vi "Create Upgrade Response.vi"(8 "error in (no error)":errorcluster, 10 "Sec-WebSocket-Key":string) -> (0 "error out":errorcluster, 2 "WebSocketUpgradeResponse":refnum<class "WebSocketUpgradeResponse.lvclass">)   [LabVIEW 2020, in "HTTP Server.lvlib" / "WebSocket Client.lvclass"]
uses:
  WebSocket Client.lvclass
  WebSocketUpgradeResponse/WebSocketUpgradeResponse.lvclass
  C:/dev/lv20CE/relink/lv-http-util/HTTP Utils/Response/Response.lvclass
  WebSocket Client.lvclass/WebSocket Client.ctl
  lv-http-util/HTTP Utils/Response/Response.lvclass
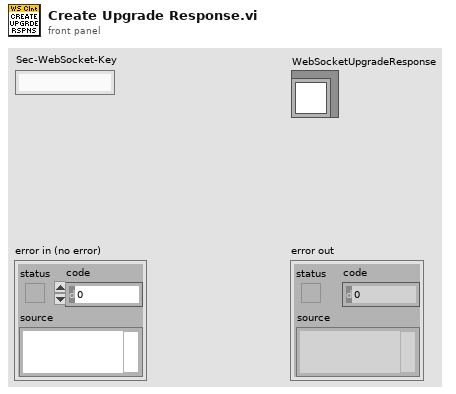
[diagram p1: front panel]
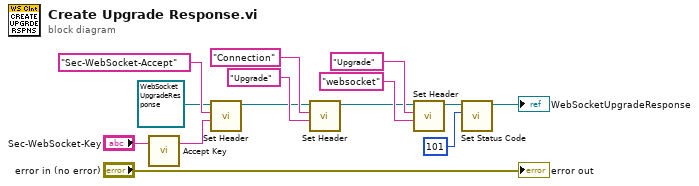
[diagram p0: block diagram]
diagram:
  n1 = call "Accept Key.vi"("Sec-WebSocket-Key"="Sec-WebSocket-Key") -> ("Sec-WebSocket-Accept"=w2:string)  [unwired: 6 in]
  n2 = call "Set Header.vi"("Value"=w2, "Header"="Sec-WebSocket-Accept", "Response in"=refnum<class "WebSocketUpgradeResponse.lvclass"> refnum ("WebSocketUpgradeResponse")) -> ("Response out"=w5:refnum<class "WebSocketUpgradeResponse.lvclass">)  [unwired: 6 in, 2 out]
  n3 = call "Set Header.vi"("Value"="Upgrade" ("Header"), "Header"="Connection", "Response in"=w5) -> ("Response out"=w7:refnum<class "WebSocketUpgradeResponse.lvclass">)  [unwired: 6 in, 2 out]
  n4 = call "Set Header.vi"("Value"="websocket" ("Header"), "Header"="Upgrade", "Response in"=w7) -> ("Response out"=w12:refnum<class "WebSocketUpgradeResponse.lvclass">)  [unwired: 6 in, 2 out]
  n5 = call "Set Status Code.vi"("Status Code"=u16 101, "Response in"=w12) -> ("Response out"=→"WebSocketUpgradeResponse":refnum<class "WebSocketUpgradeResponse.lvclass">)  [unwired: 8 in, 1 out]
  "error out" <- "error in (no error)"
